vi "Set Camera Configuration.vi"(8 "error in (no error)":errorcluster, 10 "Configuration":T1, 11 "NI Vision Camera in":refnum<class "NI Vision Camera Device.lvclass">) -> (0 "error out":errorcluster, 3 "NI Vision Camera out":refnum<class "NI Vision Camera Device.lvclass">)   [LabVIEW 2014, in "NI Vision Camera Device.lvclass"]
uses:
  NI Vision Camera Device.lvclass
  Configuration.ctl
  NI Vision Camera Device.lvclass/NI Vision Camera Device.ctl
  <resource>/objmgr/imaqdx.rc
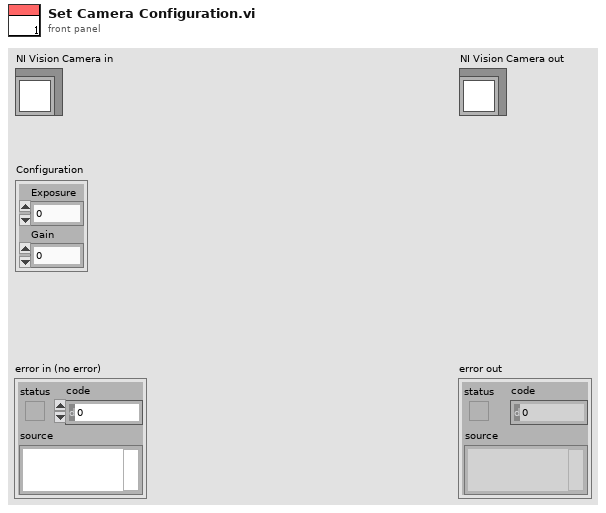
[diagram p1: front panel]
types:
  T1 = typedef "NI Vision Camera Device.lvclass/Configuration.ctl" = cluster{"Exposure":dbl, "Gain":dbl}
  T2 = typedef "IMAQdx.ctl" = refnum<k21>
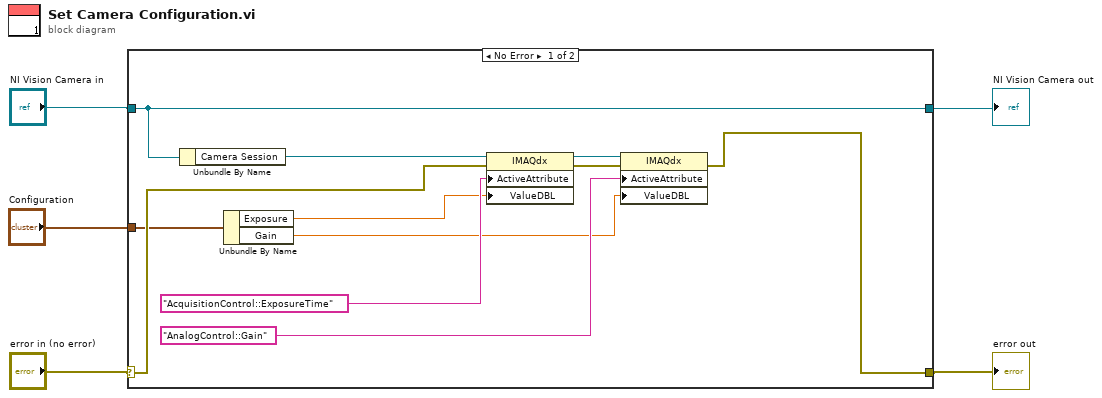
[diagram p0: block diagram]
diagram:
  n1 = case shown="No Error" "error in (no error)" {
    selector: "error in (no error)" -> [w13 w18]
    tunnel: [w7 w18] -> w4
    tunnel: [w6 w17] -> w5
    tunnel: "NI Vision Camera in" -> [w6 w17]
    tunnel: "Configuration" -> [w10 _]
    frame No Error {
      n2 = Unbundle By Name(w6) -> ("Camera Session"=w16:T2)
      n3 = Unbundle By Name(w10) -> ("Exposure"=w9:dbl, "Gain"=w8:dbl)
      n4 = property class="IMAQdx"(reference=w16, error in=w13, "ActiveAttribute"="AcquisitionControl::ExposureTime", "ValueDBL"=w9) -> (reference out=w15:T2, error out=w14:errorcluster)
      n5 = property class="IMAQdx"(reference=w15, error in=w14, "ActiveAttribute"="AnalogControl::Gain", "ValueDBL"=w8) -> (error out=w7:errorcluster)  [unwired: 1 out]
    }
    frame Error {
    }
  }
  "error out" <- w4
  "NI Vision Camera out" <- w5
